vi "Drive.vi"(0 "Robot Commands":T1, 11 "Error In":errorcluster) -> (15 "Error Out":errorcluster)   [LabVIEW 2014]
uses:
  Joystick/Robot Commands.ctl
  Global Variables/Refnum Names.vi
  <vilib>/Rock Robotics/WPI/RobotDrive/WPI_RobotDriveGetSetRefNum.vi
  <vilib>/Rock Robotics/WPI/RobotDrive/WPI_RobotDriveMecanumDrive_Cartesian.vi
  <vilib>/Rock Robotics/Network Tables/SD Write Numeric Array.vi
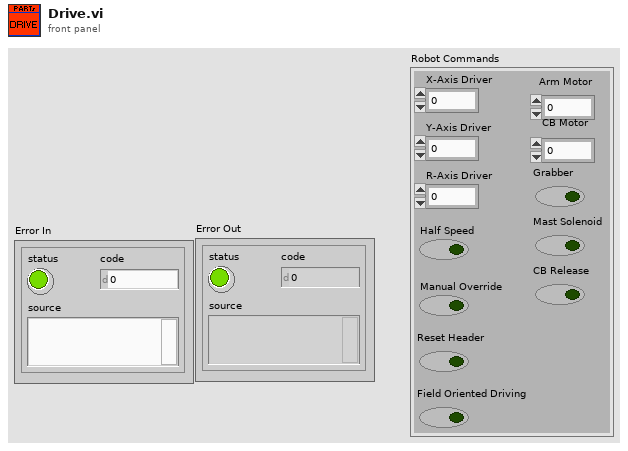
[diagram p1: front panel]
types:
  T1 = typedef "Robot Commands.ctl" = cluster{"X-Axis Driver":dbl, "Y-Axis Driver":dbl, "R-Axis Driver":dbl, "Half Speed":bool, "Manual Override":bool, "Reset Header":bool, "Field Oriented Driving":bool, "Arm Motor":dbl, "CB Motor":dbl, "Grabber":bool, "Mast Solenoid":bool, "CB Release":bool}
  T2 = typedef "WPI_RobotDriveDevRef.ctl" = cluster{"DevStatus":errorcluster, "Motors[]":T3[], "Square Inputs":bool, "Max Output":dbl}
  T3 = typedef "WPI_MotorControlDeviceRef.ctl" = cluster{"DeviceStatus":errorcluster, "Type":T4, "PWM":cluster{"Controller":T5, "PWM Channel":T6, "DeadBand":T7}, "CAN":cluster{"Device Number":u8, "Control Mode":T8, "Semaphore":T9, "Max Vout":dbl, "TalonSRX Control Mode":T10}, "Invert":bool, "TransformRef":T11, "InvTransformRef":T11}
  T4 = typedef "WPI_MotorControlType.ctl" = enum16{"PWM", "CAN", "CANTalonSRX"}
  T5 = typedef "FPGA_TypedefDigitalModule.ctl" = enum16{"Controller 1"}
  T6 = typedef "FPGA_DIOPWMChannel.ctl" = enum8{"PWM 0", "PWM 1", "PWM 2", "PWM 3", "PWM 4", "PWM 5", "PWM 6", "PWM 7", "PWM 8", "PWM 9", "PWM MXP 0", "PWM MXP 1", "PWM MXP 2", "PWM MXP 3", "PWM MXP 4", "PWM MXP 5", "PWM MXP 6", "PWM MXP 7", "PWM MXP 8", "PWM MXP 9", "Invalid"}
  T7 = typedef "WPI_PWMDeadband.ctl" = cluster{"Name":string, "maxPositivePwm":i32, "minPositivePwm":i32, "centerPwm":i32, "maxNegativePwm":i32, "minNegativePwm":i32, "angularRange":u16}
  T8 = typedef "WPI_CANJaguar_ControlMode.ctl" = enum8{"Percent VBus", "Current", "Speed", "Position", "Voltage"}
  T9 = typedef "Semaphore RefNum" = refnum<k1>
  T10 = typedef "WPI_CANTalonSRX_APIControlMode.ctl" = enum8{"Percent VBus", "Speed", "Position", "Slave", "Unchanged / Invalid"}
  T11 = typedef "WPI_PWMTransform_ConPane.ctl" = refnum<vi>
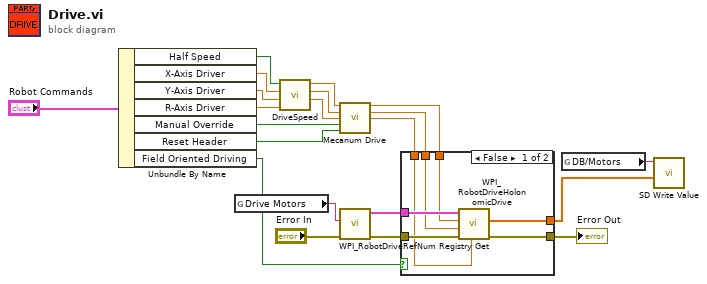
[diagram p0: block diagram]
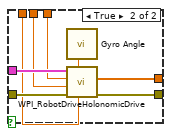
[diagram p2: hidden frame]
diagram:
  n1 = Unbundle By Name("Robot Commands") -> ("Half Speed"=w15:bool, "X-Axis Driver"=w16:dbl, "Y-Axis Driver"=w17:dbl, "R-Axis Driver"=w18:dbl, "Manual Override"=w11:bool, "Reset Header"=w10:bool, "Field Oriented Driving"=w9:bool)
  n2 = global read "Refnum Names.vi" "Drive Motors"() -> (w1:string)
  n3 = call "DriveSpeed.vi"("R In"=w18, "Y In"=w17, "X In"=w16, "Half Speed"=w15) -> ("R Out"=w12:dbl, "Y Out"=w13:dbl, "X Out"=w14:dbl)  [unwired: 5 in]
  n4 = call "Mecanum Drive.vi"("X In"=w14, "Y In"=w13, "R In"=w12, "Manual Override"=w11, "Reset Header"=w10) -> ("X Out"=w5:dbl, "Y Out"=w4:dbl, "R Out"=w3:dbl)  [unwired: 8 in]
  n5 = call <vilib>:"WPI_RobotDriveRefNum Registry Get.vi"("error in (no error)"="Error In", "refnum name"=w1) -> ("error out"=w7:errorcluster, "RobotDriveDevRef"=w8:T2)  [unwired: 8 in]
  n6 = case shown="False" w9 {
    tunnel: w8 -> [w28 w36]
    tunnel: w7 -> [w27 w35]
    tunnel: [w26 w34] -> w6
    tunnel: [w25 w33] -> w2
    tunnel: w5 -> [w24 w31]
    tunnel: w4 -> [w23 w30]
    tunnel: w3 -> [w22 w29]
    frame False {
      n7 = call-poly <vilib>:"WPI_RobotDriveHolonomicDrive.vi"("Rotation"=w22, "error in (no error)"=w27, "Y"=w23, "X"=w24, "RobotDriveDevRef"=w28) -> ("error out"=w26:errorcluster, "Motor Values"=w25:dbl[])  [unwired: 4 in, 1 out]
    }
    frame True {
      n8 = call "Gyro Angle.vi"() -> ("Angle"=w32:dbl)  [unwired: 15 in]
      n9 = call-poly <vilib>:"WPI_RobotDriveHolonomicDrive.vi"("Rotation"=w29, "Gyro Angle"=w32, "error in (no error)"=w35, "Y"=w30, "X"=w31, "RobotDriveDevRef"=w36) -> ("error out"=w34:errorcluster, "Motor Values"=w33:dbl[])  [unwired: 3 in, 1 out]
    }
  }
  "Error Out" <- w6
  n10 = global read "Refnum Names.vi" "DB/Motors"() -> (w20:string)
  n11 = call-poly <vilib>:"SD Write Value.vi"("Numeric Array"=w2, "Name"=w20) -> ()  [unwired: 8 in, 2 out]
